vi "DRAW_PATTERN_MATCHES_POSITION_ADV3(SubVI).vi"(6 "Caract. Text":T4={"Text"="", "BG Color (Transparent)"=16777216, "Text Color"=16777011, "Font, Size & Style"={"Desired Font (Application)"=enum."Application Font", "[User-specified Font]"={"Font Name"="", "Size"=12, "Strikeout?"=FALSE, "Italic?"=FALSE, "Underline?"=FALSE, "Outline?"=FALSE, "Shadow?"=FALSE, "Bold?"=FALSE, "Rotation Angle"=0.0}, "Horizontal Alignment"=0, "Vertical Alignment"=0}} {"Font, Size & Style"."Vertical Alignment" items=["Bottom", "Top", "Baseline"]; "Font, Size & Style"."Horizontal Alignment" items=["Left", "Center", "Right"]; "Font, Size & Style"."[User-specified Font]"."Rotation Angle" format="%.2f"}, 7 "color puntero":u32(colorbox)=204, 8 "Setup Show Draw":T1={"Show Text"=TRUE, "Show Center"=TRUE, "Show Bounding Box"=TRUE, "Show Angle"=FALSE}, 9 "Matches":T2(array[cluster]) {"Bounding Box"."y" format="%.2f"; "Bounding Box"."x" format="%.2f"; "Position"."y" format="%.2f"; "Position"."x" format="%.2f"; "Score" format="%.2f"; "Scale" format="%.2f"; "Angle" format="%.2f"}, 10 "Number of Matches":i32, 11 "Image Color":T3) -> (1 "Image Out":T3)   [LabVIEW 2011]
doc: "Dibuja el puntero, box, text... en un overlay de los objetos encontrados en matches.\n\nSi el numero de matches es igual a cero, no hace nada y la salida es igual a la entrada."
uses:
  IMAQ Image.ctl
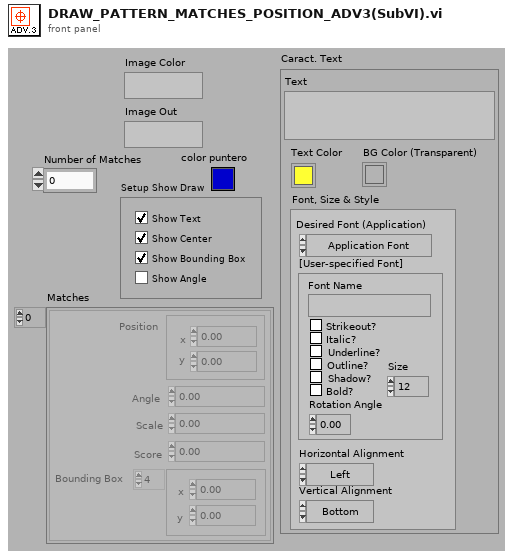
[diagram p1: front panel]
types:
  T1 = cluster{"Show Text":bool, "Show Center":bool, "Show Bounding Box":bool, "Show Angle":bool}
  T2 = cluster{"Position":cluster{"x":sgl, "y":sgl}, "Angle":sgl, "Scale":sgl, "Score":sgl, "Bounding Box":cluster{"x":sgl, "y":sgl}[]}[]
  T3 = typedef "IMAQ Image.ctl" = cluster{string, u32}
  T4 = cluster{"Text":string, "BG Color (Transparent)":u32, "Text Color":u32, "Font, Size & Style":cluster{"Desired Font (Application)":enum16{"User-specified Font", "Application Font", "System Font", "Dialog Font"}, "[User-specified Font]":cluster{"Font Name":string, "Size":i16, "Strikeout?":bool, "Italic?":bool, "Underline?":bool, "Outline?":bool, "Shadow?":bool, "Bold?":bool, "Rotation Angle":dbl}, "Horizontal Alignment":i16, "Vertical Alignment":i16}}
  T5 = cluster{"Desired Font (Application)":enum16{"User-specified Font", "Application Font", "System Font", "Dialog Font"}, "[User-specified Font]":cluster{"Font Name":string, "Size":i16, "Strikeout?":bool, "Italic?":bool, "Underline?":bool, "Outline?":bool, "Shadow?":bool, "Bold?":bool, "Rotation Angle":dbl}, "Horizontal Alignment":i16, "Vertical Alignment":i16}
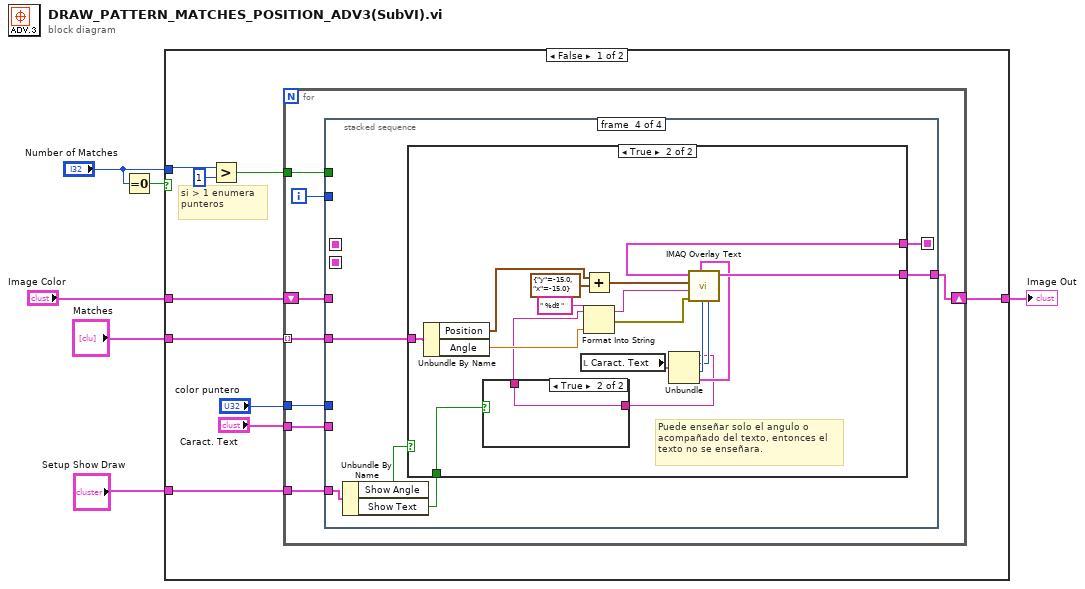
[diagram p0: block diagram]
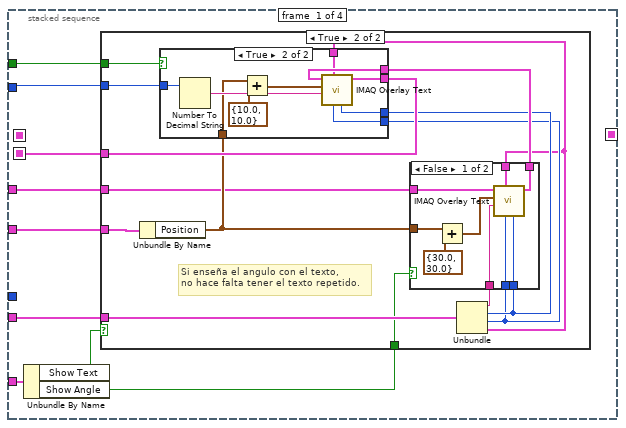
[diagram p2: hidden frame]
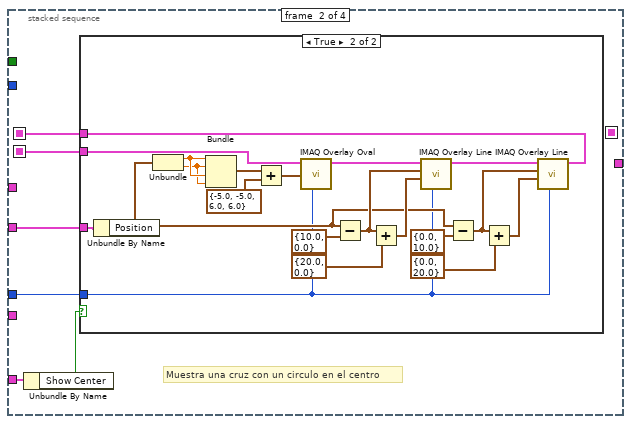
[diagram p6: hidden frame]
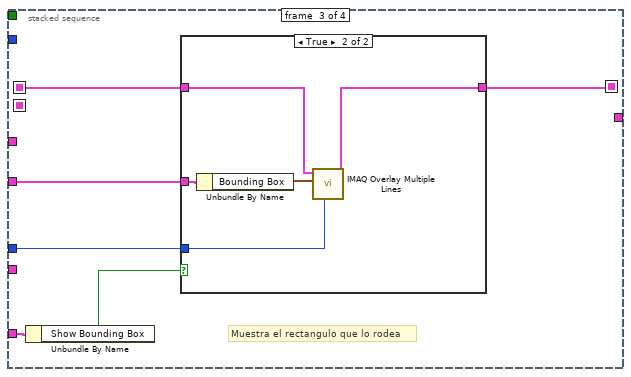
[diagram p8: hidden frame]
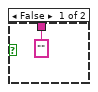
[diagram p11: hidden frame]
diagram:
  n1 = Equal To 0?(x="Number of Matches") -> (x = 0?=w5:bool)
  n2 = case shown="False" w5 {
    tunnel: "Matches" -> [w10 _]
    tunnel: [w11 w133] -> w4
    tunnel: "Image Color" -> [w12 w133]
    tunnel: "Number of Matches" -> [w15 _]
    tunnel: "Setup Show Draw" -> [w7 _]
    frame False {
      # "si > 1 enumera punteros"
      n3 = Greater?(x=w15, y=1) -> (0:w8:bool)
      n4 = for {
        shift-right: [w16] -> w11
        shift-left: w12 -> [w22]
        tunnel: w10 -> [w23] mode=indexing
        tunnel: "color puntero" -> [w21]
        tunnel: "Caract. Text" -> [w20]
        tunnel: w8 -> [w18]
        tunnel: w7 -> [w17]
        i -> [w19]
        n5 = stacked-sequence {
          seq-local: [w29 _ _ _] -> [_ w72 _ _]
          seq-local: [_ w70 _ _] -> [_ _ w99 _]
          seq-local: [_ _ w95 _] -> [_ _ _ w110]
          tunnel: w23 -> [w32 w73 w100 w108]
          tunnel: w22 -> [w26 _ _ _]
          tunnel: w21 -> [_ w71 w98 _]
          tunnel: w20 -> [w31 _ _ _]
          tunnel: w19 -> [w30 _ _ _]
          tunnel: w18 -> [w28 _ _ _]
          tunnel: w17 -> [w27 w69 w97 w112]
          tunnel: [_ _ _ w109] -> w16
          frame #0 {
            n6 = Unbundle By Name(w27) -> ("Show Text"=w25:bool, "Show Angle"=w24:bool)
            n7 = case shown="True" w25 {
              tunnel: w32 -> [_ w46]
              tunnel: w31 -> [_ w45]
              tunnel: w30 -> [_ w43]
              tunnel: [w33 w42] -> w29
              tunnel: w28 -> [_ w37]
              tunnel: w26 -> [w33 w36]
              tunnel: w24 -> [_ w35]
              frame False {
              }
              frame True {
                # "Si enseña el angulo con el texto,\nno hace falta tener el texto repetido."
                n8 = Unbundle By Name(w46) -> ("Position"=w38:cluster{"x":sgl, "y":sgl})
                n9 = Unbundle(w45) -> ("Text"=w44:string, "BG Color (Transparent)"=w40:u32, "Text Color"=w39:u32, "Font, Size & Style"=w34:T5)
                n10 = case shown="False" w35 {
                  tunnel: w44 -> [w54 _]
                  tunnel: [w53 w56] -> w41
                  tunnel: w40 -> [w51 _]
                  tunnel: w39 -> [w50 _]
                  tunnel: w38 -> [w49 _]
                  tunnel: w36 -> [w48 w56]
                  tunnel: w34 -> [w47 _]
                  frame False {
                    n11 = Add(x=w49, y=cluster{"y":sgl, "x":sgl} {"y"=30.0, "x"=30.0}) -> (x+y=w52:cluster{sgl, sgl})
                    n12 = call "IMAQ Overlay Text"("BG Color (Transparent)"=w51, "Text Color (black)"=w50, "Font, Size & Style"=w47, "String"=w54, "Origin"=w52, "Image"=w48) -> ("Image Out"=w53:T3)  [unwired: 2 in, 3 out]
                  }
                  frame True {
                  }
                }
                n13 = case shown="True" w37 {
                  tunnel: w43 -> [_ w66]
                  tunnel: [w57 w65] -> w42
                  tunnel: w41 -> [w57 w64]
                  tunnel: w38 -> [_ w61]
                  tunnel: w40 -> [_ w60]
                  tunnel: w39 -> [_ w59]
                  tunnel: w34 -> [_ w58]
                  frame False {
                  }
                  frame True {
                    n14 = Number To Decimal String(number=w66) -> (decimal integer string=w67:string)  [unwired: 1 out]
                    n15 = Add(x=w61, y=cluster{"y":sgl, "x":sgl} {"y"=10.0, "x"=10.0}) -> (x+y=w62:cluster{sgl, sgl})
                    n16 = call "IMAQ Overlay Text"("BG Color (Transparent)"=w60, "Text Color (black)"=w59, "Font, Size & Style"=w58, "String"=w67, "Origin"=w62, "Image"=w64) -> ("Image Out"=w65:T3)  [unwired: 2 in, 3 out]
                  }
                }
              }
            }
          }
          frame #1 {
            # "Muestra una cruz con un circulo en el centro"
            n17 = Unbundle By Name(w69) -> ("Show Center"=w68:bool)
            n18 = case shown="True" w68 {
              tunnel: w73 -> [_ w94]
              tunnel: w72 -> [w74 w82]
              tunnel: w71 -> [_ w75]
              tunnel: [w74 w85] -> w70
              frame False {
              }
              frame True {
                n19 = Unbundle By Name(w94) -> ("Position"=w76:cluster{"x":sgl, "y":sgl})
                n20 = Unbundle(w76) -> ("x"=w81:sgl, "y"=w80:sgl)
                n21 = Bundle("x"=w81, "y"=w80, "x"=w81, "y"=w80) -> (w79:cluster{"x":sgl, "y":sgl, "x":sgl, "y":sgl})  [unwired: 1 out]
                n22 = Add(x=w79, y=cluster{"y":sgl, "x":sgl, "y":sgl, "x":sgl} {"y"=-5.0, "x"=-5.0, "y"=6.0, "x"=6.0}) -> (x+y=w77:cluster{sgl, sgl, sgl, sgl})
                n23 = call "IMAQ Overlay Oval"("Color"=w75, "Bounding Rectangle"=w77, "Image"=w82) -> ("Image Out"=w83:T3)  [unwired: 3 in, 5 out]
                n24 = Subtract(x=w76, y=cluster{"x":sgl, "y":sgl} {"x"=10.0, "y"=0.0}) -> (x-y=w92:cluster{"x":sgl, "y":sgl})
                n25 = Add(x=w92, y=cluster{"x":sgl, "y":sgl} {"x"=20.0, "y"=0.0}) -> (x+y=w90:cluster{"x":sgl, "y":sgl})
                n26 = call "IMAQ Overlay Line"("Color"=w75, "End Point"=w90, "Start Point"=w92, "Image"=w83) -> ("Image Out"=w84:T3)  [unwired: 2 in, 5 out]
                n27 = Subtract(x=w76, y=cluster{"x":sgl, "y":sgl} {"x"=0.0, "y"=10.0}) -> (x-y=w88:cluster{"x":sgl, "y":sgl})
                n28 = Add(x=w88, y=cluster{"x":sgl, "y":sgl} {"x"=0.0, "y"=20.0}) -> (x+y=w89:cluster{"x":sgl, "y":sgl})
                n29 = call "IMAQ Overlay Line"("Color"=w75, "End Point"=w89, "Start Point"=w88, "Image"=w84) -> ("Image Out"=w85:T3)  [unwired: 2 in, 5 out]
              }
            }
          }
          frame #2 {
            # "Muestra el rectangulo que lo rodea"
            n30 = Unbundle By Name(w97) -> ("Show Bounding Box"=w96:bool)
            n31 = case shown="True" w96 {
              tunnel: w100 -> [_ w106]
              tunnel: w99 -> [w101 w105]
              tunnel: [w101 w104] -> w95
              tunnel: w98 -> [_ w103]
              frame False {
              }
              frame True {
                n32 = Unbundle By Name(w106) -> ("Bounding Box"=w102:cluster{"x":sgl, "y":sgl}[])
                n33 = call "IMAQ Overlay Multiple Lines"("Color"=w103, "Line End Points"=w102, "Image"=w105) -> ("Image Out"=w104:T3)  [unwired: 3 in, 5 out]
              }
            }
          }
          frame #3 {
            n34 = Unbundle By Name(w112) -> ("Show Angle"=w111:bool, "Show Text"=w107:bool)
            n35 = case shown="True" w111 {
              tunnel: w110 -> [w113 w130]
              tunnel: [w113 w129] -> w109
              tunnel: w108 -> [_ w128]
              tunnel: w107 -> [_ w116]
              frame False {
              }
              frame True {
                # "Puede enseñar solo el angulo o\nacompañado del texto, entonces el\ntexto no se enseñara."
                n36 = Unbundle By Name(w128) -> ("Position"=w120:cluster{"x":sgl, "y":sgl}, "Angle"=w119:sgl)
                n37 = local read "Caract. Text"() -> (w125:T4)
                n38 = Add(x=w120, y=cluster{"y":sgl, "x":sgl} {"y"=-15.0, "x"=-15.0}) -> (x+y=w123:cluster{sgl, sgl})
                n39 = Unbundle(w125) -> ("Text"=w114:string, "BG Color (Transparent)"=w117:u32, "Text Color"=w118:u32, "Font, Size & Style"=w124:T5)
                n40 = case shown="True" w116 {
                  tunnel: ["" ("Text") w132] -> w115
                  tunnel: w114 -> [_ w132]
                  frame False {
                  }
                  frame True {
                  }
                }
                n41 = Format Into String(format string=" %dº ", initial string=w115, w119) -> (resulting string=w126:string, error out=w122:errorcluster)  [unwired: 1 in]
                n42 = call "IMAQ Overlay Text"("BG Color (Transparent)"=w117, "Text Color (black)"=w118, "Font, Size & Style"=w124, "error in (no error)"=w122, "String"=w126, "Origin"=w123, "Image"=w130) -> ("Image Out"=w129:T3)  [unwired: 1 in, 3 out]
              }
            }
          }
        }
      }
    }
    frame True {
    }
  }
  "Image Out" <- w4
